vi "escape string performance.vi"() -> ()   [LabVIEW 2013]
uses:
  JSONtext.lvlib
panel:
  in  "cut down to length":i32=10000
  out "escaped len":i32
  out "cut down length":i32
  out "x = y?":bool[](array[boolean])
  in  "unicode":bool=TRUE
  out "Array 2":string[](array[string])
  out "t":dbl[](array[numeric])=[0.2729243521175704, 0.3112940331802747, 1.583932036054648, 0.303617638554897]
  # "lvjson"
  # "ds"
  # "jsontxt"
  # "ds w/ conditional\nunicode"
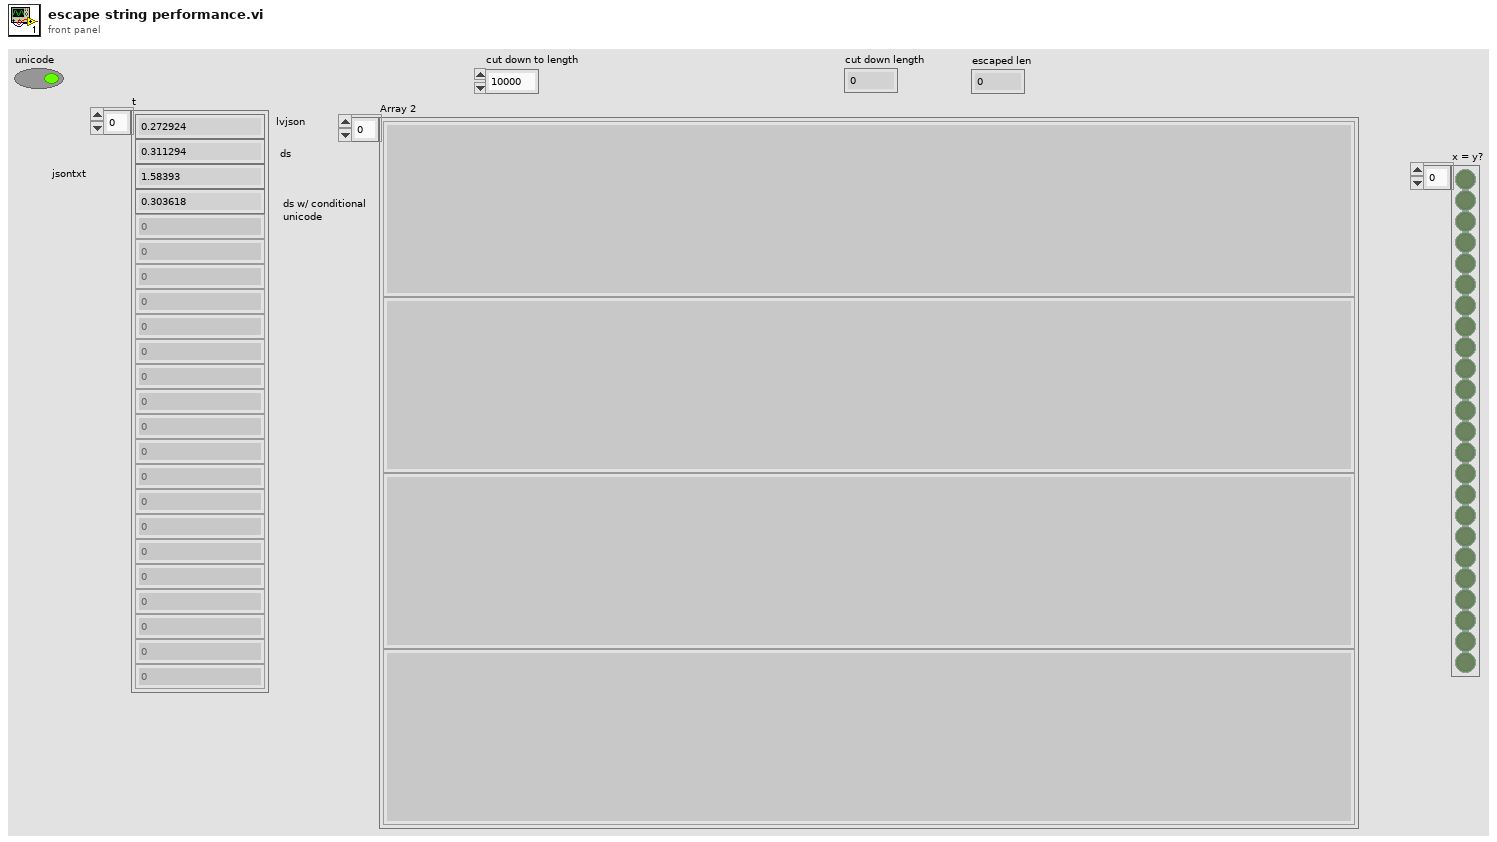
[diagram p1: front panel]
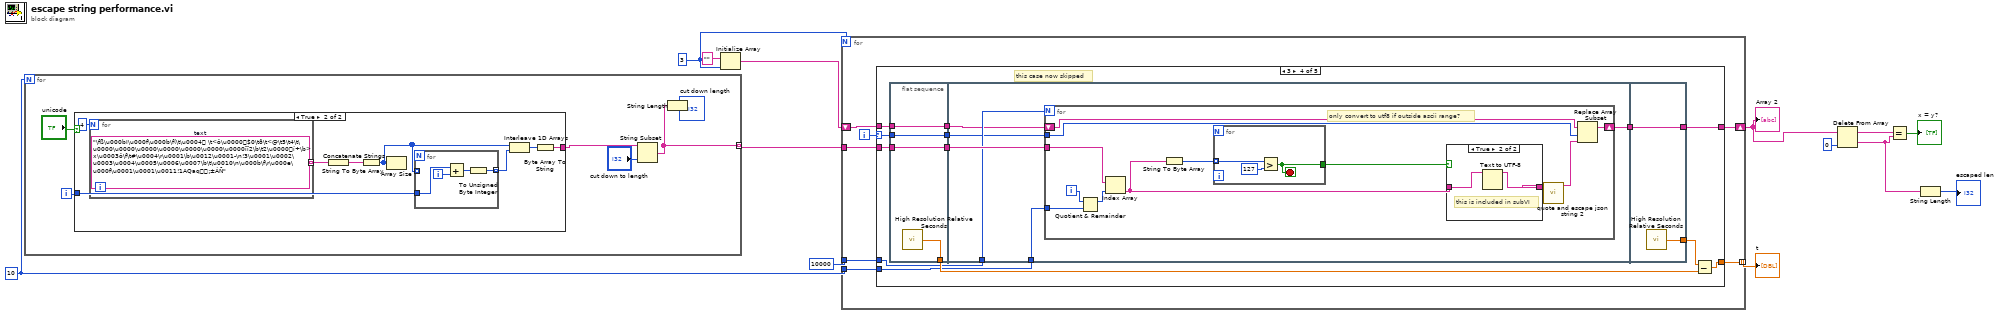
[diagram p0: block diagram]
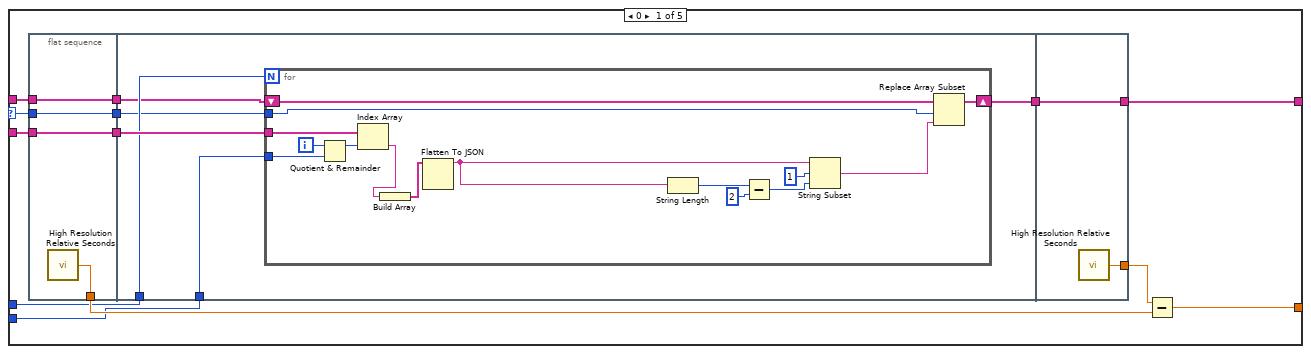
[diagram p2: hidden frame]
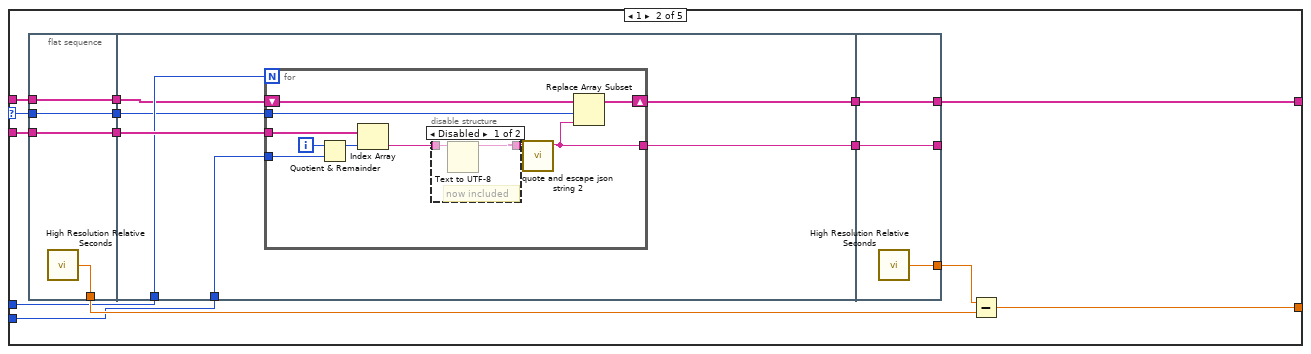
[diagram p3: hidden frame]
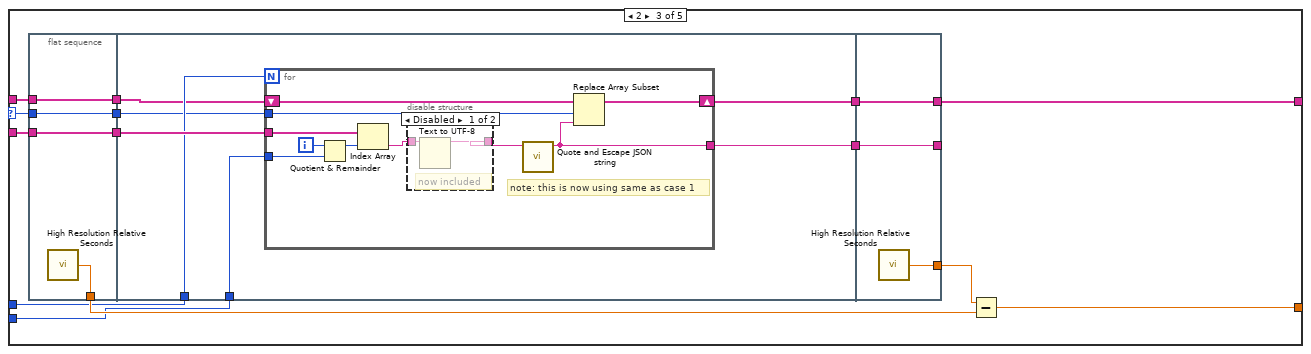
[diagram p5: hidden frame]
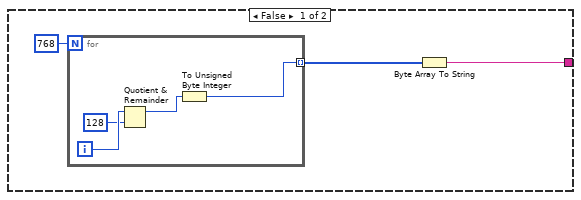
[diagram p9: hidden frame]
diagram:
  w8 = 3
  w12 = 10
  n1 = for {
    N: w12 -> [_]
    tunnel: [w14] -> w10 mode=indexing
    i -> [w19]
    n2 = case shown="True" "unicode" {
      tunnel: w19 -> [_ w33]
      tunnel: [w20 w29] -> w17
      frame False {
        n3 = for {
          N: 768 -> [_]
          tunnel: [w23] -> w21 mode=indexing
          i -> [w26]
          n4 = Quotient & Remainder(x=w26, y=128) -> (x-y*floor(x/y)=w24:i32)  [unwired: 1 out]
          n5 = To Unsigned Byte Integer(number=w24) -> (unsigned 8bit integer=w23:u8)
        }
        n6 = Byte Array To String(unsigned byte array=w21) -> (string=w20:string)
      }
      frame True {
        n7 = for {
          N: 4 -> [_]
          tunnel: [w35] -> w34 mode=indexing
          w35 = "\fß\u000bI\u000f\u000b\f(\t\u0004 \t<ô\u0000$0\tð\t<@\t5\t4\t\u0000\u0000\u0000\u0000\u0000\u0000\u0000ïï2\b\t2\u0000í÷\b> x\u0003ô\f\t#\u0004\r\u0001\b\u0012\u0001-\n!3\u0001\u0002\u0003\u0004\u0005\u0006\u0007\b\t\u0010\n\u000b\f\r\u000e\u000f\u0001\u0001\u0011!1AQaq¡±ÁÑ"  # text
        }
        n8 = Concatenate Strings(w34) -> (w27:string)
        n9 = String To Byte Array(string=w27) -> (unsigned byte array=w31:u8[])
        n10 = Array Size(array=w31) -> ()  [unwired: 1 out]
        n11 = for {
          tunnel: w31 -> [_] mode=indexing
          tunnel: w33 -> [w38]
          tunnel: [w36] -> w32 mode=indexing
          i -> [w39]
          n12 = Add(x=w38, y=w39) -> (x+y=w37:i32)
          n13 = To Unsigned Byte Integer(number=w37) -> (unsigned 8bit integer=w36:u8)
        }
        n14 = Interleave 1D Arrays(w31, w32) -> (w30:u8[])
        n15 = Byte Array To String(unsigned byte array=w30) -> (string=w29:string)
      }
    }
    n16 = String Subset(string=w17, length (rest)="cut down to length") -> (substring=w14:string)  [unwired: 1 in]
    n17 = String Length(string=w14) -> (length=→"cut down length":i32)
  }
  n18 = Initialize Array("", w8) -> (w7:string[])
  n19 = for {
    N: w8 -> [_]
    tunnel: w10 -> [w44]
    tunnel: [w45] -> w13 mode=indexing
    tunnel: w12 -> [w43]
    tunnel: 10000 -> [w42]
    shift-right: [w40] -> w6
    shift-left: w7 -> [w41]
    i -> [w46]
    n20 = case shown="3" w46 {
      selector: w46 -> [w48 w88 w129 w170 _]
      tunnel: [w57 w98 w139 w179 _] -> w45
      tunnel: w44 -> [w55 w96 w137 w177 _]
      tunnel: w43 -> [w54 w95 w136 w176 _]
      tunnel: w42 -> [w53 w94 w135 w175 _]
      tunnel: w41 -> [w52 w92 w133 w174 w212]
      tunnel: [w50 w90 w131 w172 w212] -> w40
      frame 0 {
        n21 = flat-sequence {
          tunnel: [w63] -> w58
          tunnel: [w62] -> w56
          tunnel: w55 -> [w62]
          tunnel: w52 -> [w61]
          tunnel: [w61] -> w51
          tunnel: w48 -> [w60]
          tunnel: [w60] -> w47
          tunnel: w56 -> [w68]
          tunnel: w54 -> [w69]
          tunnel: w53 -> [w67]
          tunnel: w51 -> [w66]
          tunnel: [w65] -> w49
          tunnel: w47 -> [w64]
          tunnel: [w86] -> w59
          tunnel: [w85] -> w50
          tunnel: w49 -> [w85]
          frame #0 {
            n22 = call <vilib>:"High Resolution Relative Seconds.vi"() -> ("relative seconds"=w63:dbl)
          }
          frame #1 {
            n23 = for {
              N: w67 -> [_]
              tunnel: w69 -> [w83]
              tunnel: w68 -> [w81]
              shift-right: [w79] -> w65
              shift-left: w66 -> [w80]
              tunnel: w64 -> [w78]
              i -> [w84]
              n24 = Quotient & Remainder(x=w84, y=w83) -> (x-y*floor(x/y)=w82:i32)  [unwired: 1 out]
              n25 = Index Array(array=w81, index=w82) -> (element=w71:string)
              n26 = Build Array(w71) -> (w77:string[])
              n27 = Flatten To JSON(anything=w77) -> (JSON string=w75:string)  [unwired: 2 in, 1 out]
              n28 = String Length(string=w75) -> (length=w74:i32)
              n29 = Subtract(x=w74, y=2) -> (x-y=w72:i32)
              n30 = String Subset(string=w75, offset (0)=1, length (rest)=w72) -> (substring=w70:string)
              n31 = Replace Array Subset(array=w80, new element=w70, index=w78) -> (w79:string[])
            }
          }
          frame #2 {
            n32 = call <vilib>:"High Resolution Relative Seconds.vi"() -> ("relative seconds"=w86:dbl)
          }
        }
        n33 = Subtract(x=w59, y=w58) -> (x-y=w57:dbl)
      }
      frame 1 {
        n34 = flat-sequence {
          tunnel: [w104] -> w99
          tunnel: [w103] -> w97
          tunnel: w96 -> [w103]
          tunnel: w92 -> [w102]
          tunnel: [w102] -> w91
          tunnel: w88 -> [w101]
          tunnel: [w101] -> w87
          tunnel: w97 -> [w110]
          tunnel: w95 -> [w111]
          tunnel: w94 -> [w109]
          tunnel: [w108] -> w93
          tunnel: w91 -> [w107]
          tunnel: [w106] -> w89
          tunnel: w87 -> [w105]
          tunnel: [w127] -> w100
          tunnel: [w126] -> _
          tunnel: w93 -> [w126]
          tunnel: [w125] -> w90
          tunnel: w89 -> [w125]
          frame #0 {
            n35 = call <vilib>:"High Resolution Relative Seconds.vi"() -> ("relative seconds"=w104:dbl)
          }
          frame #1 {
            n36 = for {
              N: w109 -> [_]
              tunnel: w111 -> [w120]
              tunnel: w110 -> [w118]
              tunnel: [w112] -> w108
              shift-right: [w116] -> w106
              shift-left: w107 -> [w117]
              tunnel: w105 -> [w115]
              i -> [w121]
              n37 = Quotient & Remainder(x=w121, y=w120) -> (x-y*floor(x/y)=w119:i32)  [unwired: 1 out]
              n38 = Index Array(array=w118, index=w119) -> (element=w114:string)
              n39 = disable-structure shown="Disabled" {
                disable-tunnel: w114 -> [w123 w124]
                disable-tunnel: [w122 w124] -> w113
                frame Disabled {
                  # "now included"
                  n40 = Text to UTF-8(11:w123) -> (3:w122:string)  [unwired: 1 in, 1 out]
                }
                frame Enabled {
                }
              }
              n41 = call "quote and escape json string 2.vi"("base string"=w113) -> ("String out"=w112:string)  [unwired: 10 in]
              n42 = Replace Array Subset(array=w117, new element=w112, index=w115) -> (w116:string[])
            }
          }
          frame #2 {
            n43 = call <vilib>:"High Resolution Relative Seconds.vi"() -> ("relative seconds"=w127:dbl)
          }
        }
        n44 = Subtract(x=w100, y=w99) -> (x-y=w98:dbl)
      }
      frame 2 {
        n45 = flat-sequence {
          tunnel: [w145] -> w140
          tunnel: [w144] -> w138
          tunnel: w137 -> [w144]
          tunnel: w133 -> [w143]
          tunnel: [w143] -> w132
          tunnel: w129 -> [w142]
          tunnel: [w142] -> w128
          tunnel: w138 -> [w151]
          tunnel: w136 -> [w152]
          tunnel: w135 -> [w150]
          tunnel: [w149] -> w134
          tunnel: w132 -> [w148]
          tunnel: [w147] -> w130
          tunnel: w128 -> [w146]
          tunnel: [w168] -> w141
          tunnel: [w167] -> _
          tunnel: w134 -> [w167]
          tunnel: [w166] -> w131
          tunnel: w130 -> [w166]
          frame #0 {
            n46 = call <vilib>:"High Resolution Relative Seconds.vi"() -> ("relative seconds"=w145:dbl)
          }
          frame #1 {
            n47 = for {
              N: w150 -> [_]
              tunnel: w152 -> [w161]
              tunnel: w151 -> [w159]
              tunnel: [w153] -> w149
              shift-right: [w157] -> w147
              shift-left: w148 -> [w158]
              tunnel: w146 -> [w156]
              i -> [w162]
              # "note: this is now using same as case 1"
              n48 = Quotient & Remainder(x=w162, y=w161) -> (x-y*floor(x/y)=w160:i32)  [unwired: 1 out]
              n49 = Index Array(array=w159, index=w160) -> (element=w155:string)
              n50 = disable-structure shown="Disabled" {
                disable-tunnel: w155 -> [w164 w165]
                disable-tunnel: [w163 w165] -> w154
                frame Disabled {
                  # "now included"
                  n51 = Text to UTF-8(11:w164) -> (3:w163:string)  [unwired: 1 in, 1 out]
                }
                frame Enabled {
                }
              }
              n52 = call "Quote and Escape JSON string.vi"("Plain Text"=w154) -> ("<JSON>"=w153:string)  [unwired: 10 in]
              n53 = Replace Array Subset(array=w158, new element=w153, index=w156) -> (w157:string[])
            }
          }
          frame #2 {
            n54 = call <vilib>:"High Resolution Relative Seconds.vi"() -> ("relative seconds"=w168:dbl)
          }
        }
        n55 = Subtract(x=w141, y=w140) -> (x-y=w139:dbl)
      }
      frame 3 {
        # "this case now skipped"
        n56 = flat-sequence {
          tunnel: [w185] -> w180
          tunnel: [w184] -> w178
          tunnel: w177 -> [w184]
          tunnel: w174 -> [w183]
          tunnel: [w183] -> w173
          tunnel: w170 -> [w182]
          tunnel: [w182] -> w169
          tunnel: w178 -> [w190]
          tunnel: w176 -> [w191]
          tunnel: w175 -> [w189]
          tunnel: w173 -> [w188]
          tunnel: [w187] -> w171
          tunnel: w169 -> [w186]
          tunnel: [w211] -> w181
          tunnel: [w210] -> w172
          tunnel: w171 -> [w210]
          frame #0 {
            n57 = call <vilib>:"High Resolution Relative Seconds.vi"() -> ("relative seconds"=w185:dbl)
          }
          frame #1 {
            n58 = for {
              N: w189 -> [_]
              tunnel: w191 -> [w202]
              tunnel: w190 -> [w200]
              shift-right: [w198] -> w187
              shift-left: w188 -> [w199]
              tunnel: w186 -> [w197]
              i -> [w203]
              # "only convert to utf8 if outside ascii range?"
              n59 = Quotient & Remainder(x=w203, y=w202) -> (x-y*floor(x/y)=w201:i32)  [unwired: 1 out]
              n60 = Index Array(array=w200, index=w201) -> (element=w194:string)
              n61 = String To Byte Array(string=w194) -> (unsigned byte array=w196:u8[])
              n62 = for {
                tunnel: w196 -> [w209] mode=indexing
                tunnel: [w207] -> w195
                stop <- w207 stop-if-true
                n63 = Greater?(x=w209, y=u8 127) -> (0:w207:bool)
              }
              n64 = case shown="True" w195 {
                tunnel: [w204 w206] -> w193
                tunnel: w194 -> [w204 w205]
                frame False {
                }
                frame True {
                  # "this is included in subVI"
                  n65 = Text to UTF-8(11:w205) -> (3:w206:string)  [unwired: 1 in, 1 out]
                }
              }
              n66 = call "quote and escape json string 2.vi"("base string"=w193) -> ("String out"=w192:string)  [unwired: 10 in]
              n67 = Replace Array Subset(array=w199, new element=w192, index=w197) -> (w198:string[])
            }
          }
          frame #2 {
            n68 = call <vilib>:"High Resolution Relative Seconds.vi"() -> ("relative seconds"=w211:dbl)
          }
        }
        n69 = Subtract(x=w181, y=w180) -> (x-y=w179:dbl)
      }
      frame Default {
      }
    }
  }
  "t" <- w13
  "Array 2" <- w6
  n70 = Delete From Array(array=w6, index=0) -> (deleted portion=w1:string, array with subset deleted=w3:string[])  [unwired: 1 in]
  n71 = Equal?(x=w3, y=w1) -> (x = y?=→"x = y?":bool[])
  n72 = String Length(string=w1) -> (length=→"escaped len":i32)
